vi "ATF Pumb-RT_Main.vi"   [LabVIEW 2022 SP3]
uses:
  RT Controls/RT main.ctl
  RT Support/SeCrTs-RT_Global_R.vi
panel:
  # "RT main ATF-Pump"
types:
  T1 = typedef "RT main.ctl" = enum16{"initialise", "Wait for connection", "Wait for command"}
  T2 = enum16{"Init", "Read 'All'", "Read 'n'", "Read '1'", "Write '1'", "Write 'n'", "Write 'All'"}
  T3 = cluster{"Drive Control":cluster{"En_Drive_A":bool, "En_Drive_L":bool, "Exit_Drive_A":bool, "Exit_Drive_L":bool}, "Drive_ATF Control":cluster{"S.Freq":dbl, "Ramp up Time":dbl, "Ramp down Time":dbl, "Drive Speed":dbl, "Drive condition":dbl}, "Drive_LOX Control":cluster{"S.Freq":dbl, "Ramp up Time":dbl, "Ramp down Time":dbl, "Drive Speed":dbl, "Drive condition":dbl}, "Aconnection ID":refnum<k5>, "Lconnection ID":refnum<k5>, "Loop Control":cluster{"Start DAQ":bool, "Stop DAQ":bool, "RT Stop":bool, "RT Exit":bool, "Start Seq":bool}}
  T4 = typedef "SeCrTs-Data FIFO.ctl" = cluster{"RD":cluster{"AI_V_Data RD":refnum<queue>, "AI_C_Data RD":refnum<queue>, "AO_Data RD":refnum<queue>, "DI_Data RD":refnum<queue>, "ACC_Data RD":refnum<queue>, "TC_Data RD":refnum<queue>, "Drive_A_C RD":refnum<queue>, "Drive_A_D RD":refnum<queue>, "Drive_L_C RD":refnum<queue>, "Drive_L_D RD":refnum<queue>, "DI Data":refnum<queue>, "DO_Data RD":refnum<queue>}, "Err Pump":refnum<queue>}
  T5 = cluster{"Device List":cluster{"AO Cards":tag[], "AI Cards":tag[], "DI Cards":tag[], "DO Cards":tag[]}, "Channel List":cluster{"AI Channel list":tag[], "AO Channel list":tag[], "DO Channel list ":tag[], "DI Channel list":tag[]}}
  T6 = cluster{cluster{"Sr. No.":string, "Time CDT":string, "Component ID":string, "Data Type":string, "Condition":string, "Range/Position":string, "No of Samples for Pass":string, "Event Duration":string, "Continuous /Cumulative":string, "Expected Delay":string, "Failure case Seq":string, "Current Sequence":string}[]}[]
  T7 = cluster{"AO config":cluster{"Channel_Name":string, "Channel_Number":string, "Default_Value":dbl, "Units":string}[], "AI config":cluster{"Channel_Name":string, "Channel_Number":string, "Pre_Scale_min":dbl, "Pre_Scale_max":dbl, "Sensor_min":dbl, "Sensor_max":dbl, "Units":string}[], "DI config":cluster{"Channel_Name":string, "Channel_Number":string, "Default_Value":bool, "DI invert?":bool}[], "DO config":cluster{"Channel_Name":string, "Channel_Number":string, "Default_Value":bool, "DO invert?":bool}[], "TC config":cluster{"Channel_Name":string, "Channel_Number":string, "Pre_Scale_min":dbl, "Pre_Scale_max":dbl, "units":i32, " type":i32}[], "ACC config":cluster{"Channel_Name":string, "Channel_Number":string, "Pre_Scale_min":dbl, "Pre_Scale_max":dbl, "Terminal configuration":i32, "Sensitivity":dbl, "Sensitivity units":i32}[], "SG config":cluster{"Channel_Name":string, "Channel_Number":string, "Pre_Scale_min":dbl, "Pre_Scale_max":dbl}[], "Strain Gauge Settings":cluster{"poisson ratio":dbl, "nominal gage resistance":dbl, "gage factor":dbl}, "Bridge Settings":cluster{"voltage excitation value":dbl, "voltage excitation source":i32, "initial bridge voltage":dbl, "lead wire resistance":dbl, "strain configuration":i32}, "Sample Rate":cluster{"AI Sample Rate":dbl[], "AO Sample Rate":dbl[], "DI Sample Rate":dbl[], "TC Sample Rate":dbl[], "DO Sample Rate":dbl[], "SG Sample Rate":dbl[], "ACC Sample Rate":dbl[]}}
  T8 = enum16{"Init", "Read", "Write 'All'", "Write 'n'", "Write Safe Value", "Write Start Time", "Overwrite Pattern", "Overwrite Pattern with Start", "Append Pattern", "Start Pattern Mode", "Abort Pattern Mode", "Read 1"}
  T9 = cluster{"S.Freq":dbl, "Ramp up Time":dbl, "Ramp down Time":dbl, "Drive Speed":dbl, "Drive condition":dbl}
  T10 = cluster{"AO Cards":tag[], "AI Cards":tag[], "DI Cards":tag[], "DO Cards":tag[]}
  T11 = cluster{"AI Channel list":tag[], "AO Channel list":tag[], "DO Channel list ":tag[], "DI Channel list":tag[]}
  T12 = cluster{"Start DAQ":bool, "Stop DAQ":bool, "RT Stop":bool, "RT Exit":bool, "Start Seq":bool}
  T13 = cluster{"En_Drive_A":bool, "En_Drive_L":bool, "Exit_Drive_A":bool, "Exit_Drive_L":bool}
  T14 = cluster{"Manual HOLD":bool, "Automatic Hold AI":bool, "Abort":bool, "Automatic Hold DI":bool}
  T15 = cluster{"Channel_Name":string, "Channel_Number":string, "Default_Value":bool, "DO invert?":bool}[]
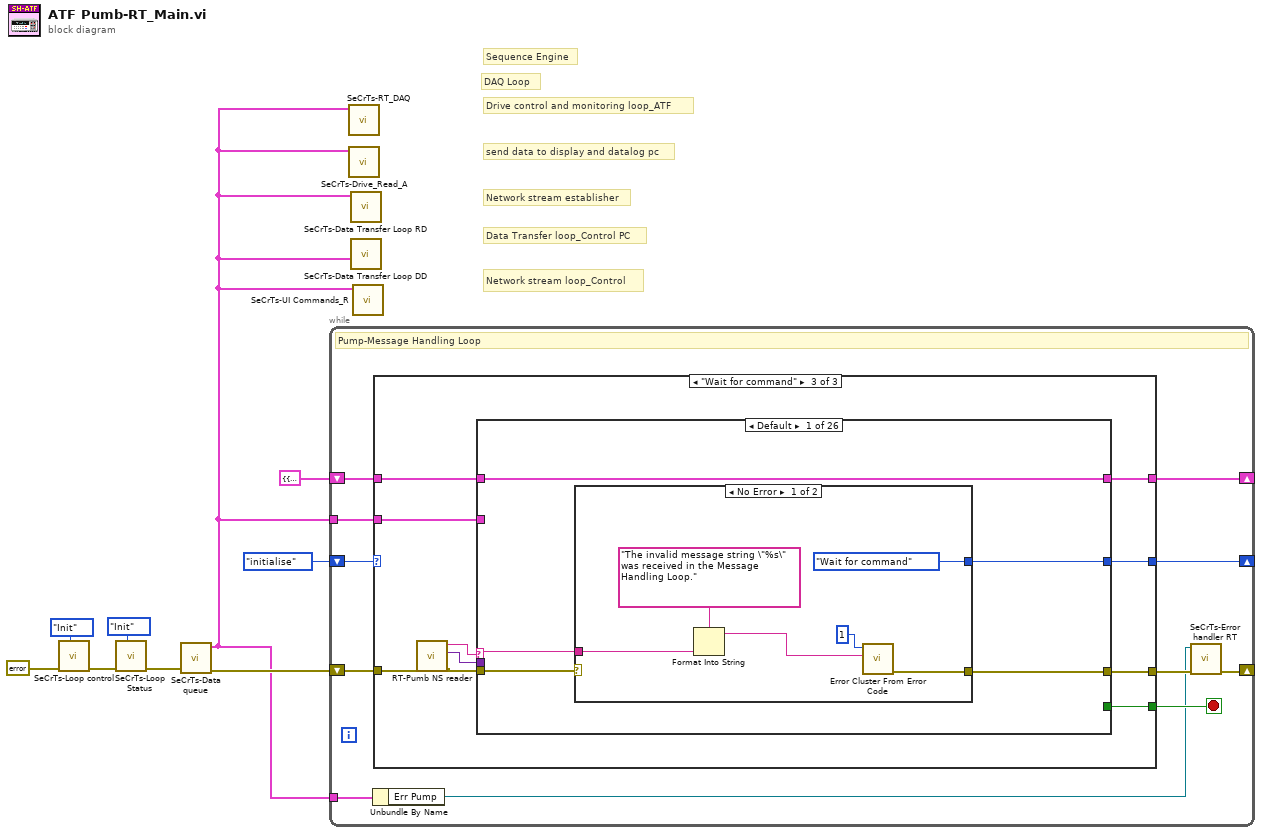
[diagram p0: block diagram]
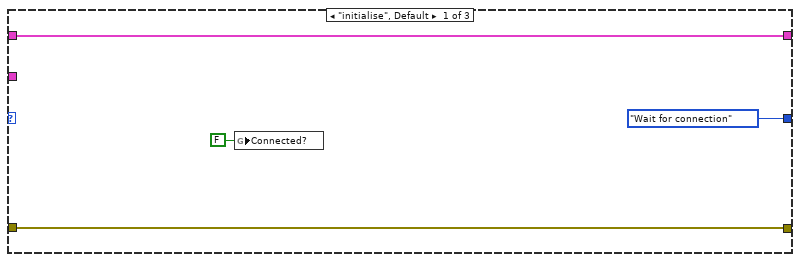
[diagram p2: hidden frame]
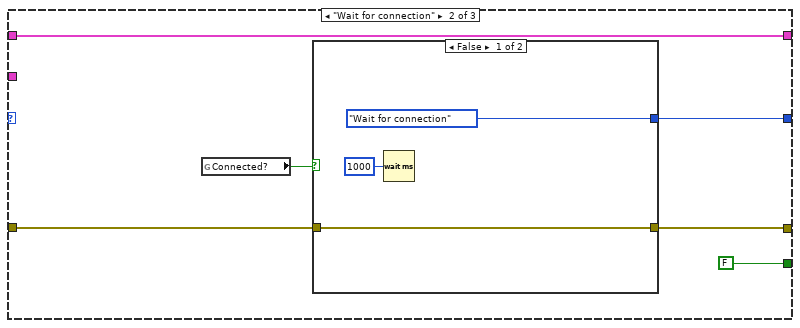
[diagram p3: hidden frame]
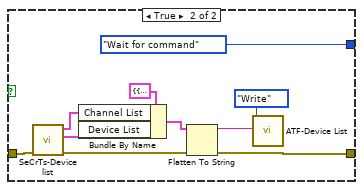
[diagram p4: hidden frame]
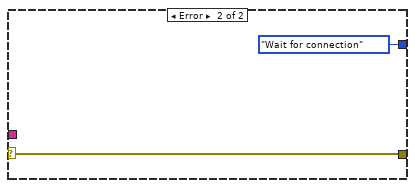
[diagram p5: hidden frame]
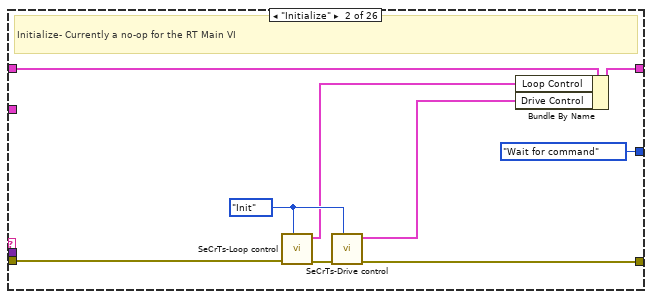
[diagram p6: hidden frame]
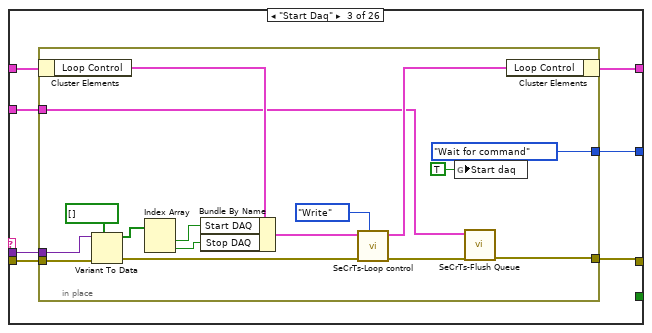
[diagram p7: hidden frame]
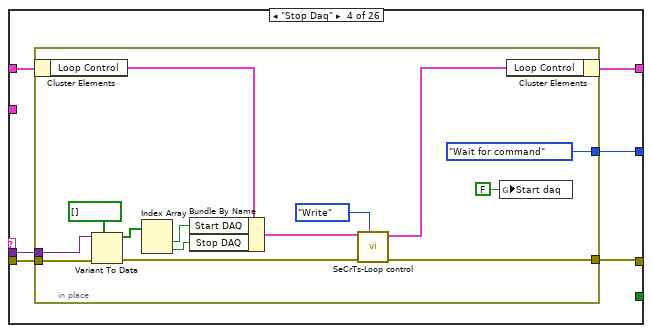
[diagram p8: hidden frame]
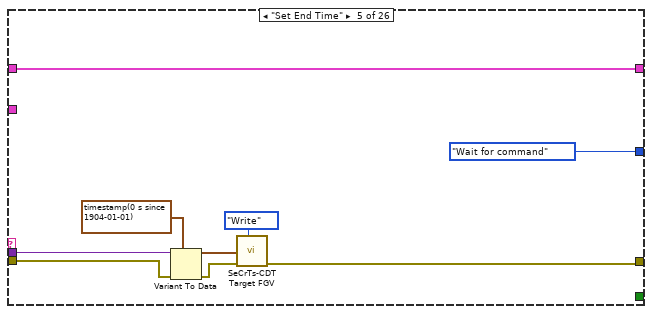
[diagram p9: hidden frame]
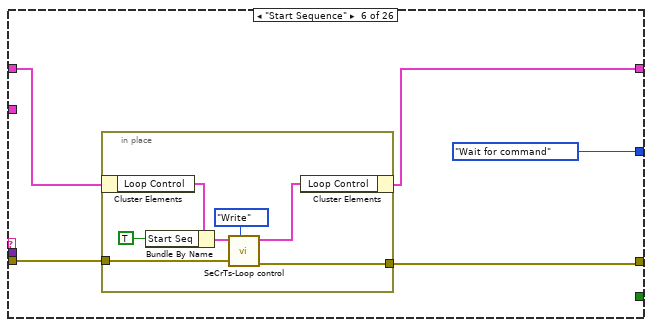
[diagram p10: hidden frame]
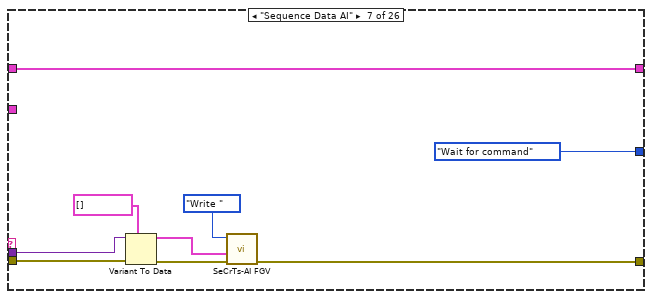
[diagram p11: hidden frame]
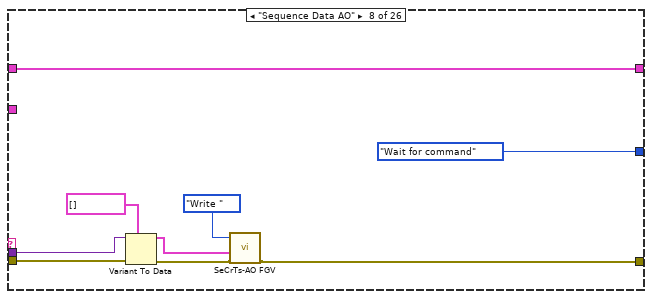
[diagram p12: hidden frame]
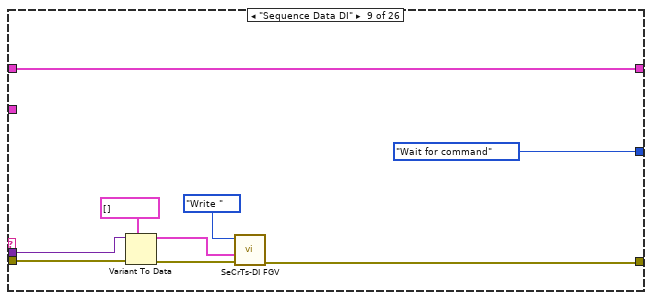
[diagram p13: hidden frame]
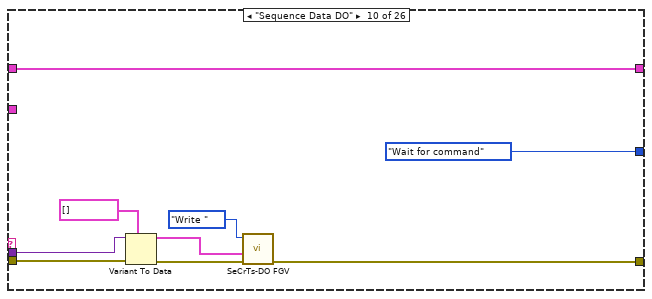
[diagram p14: hidden frame]
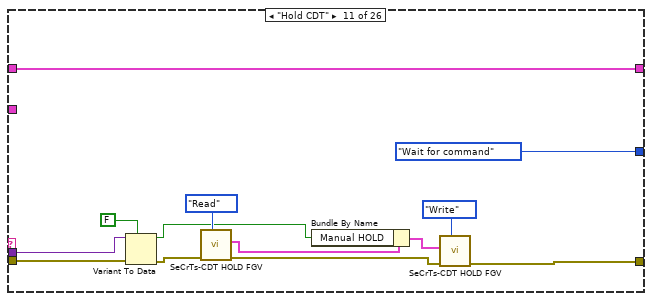
[diagram p15: hidden frame]
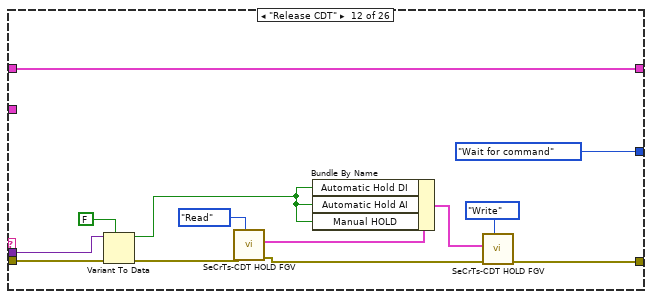
[diagram p16: hidden frame]
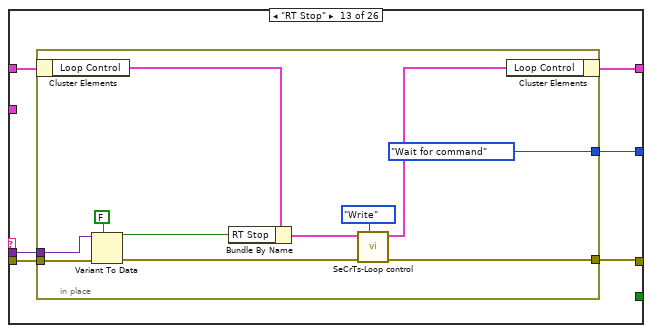
[diagram p17: hidden frame]
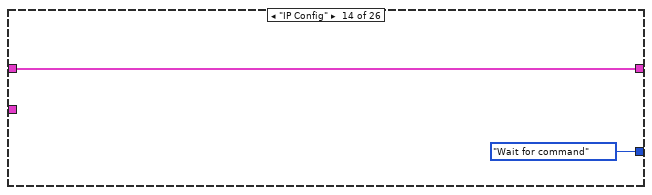
[diagram p18: hidden frame]
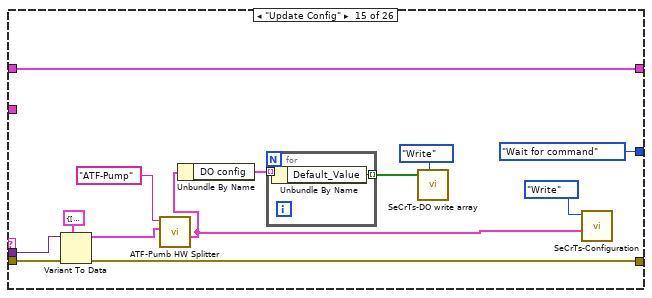
[diagram p19: hidden frame]
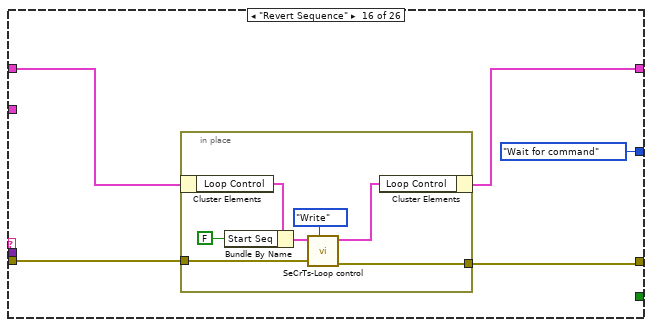
[diagram p20: hidden frame]
diagram:
  # "Sequence Engine"
  # "send data to display and datalog pc"
  # "Network stream establisher"
  # "Data Transfer loop_Control PC"
  # "Drive control and monitoring loop_ATF"
  # "DAQ Loop"
  # "Network stream loop_Control"
  n1 = call "SeCrTs-Loop control.vi"("Action"=enum16{"Init", "Write", "Read"}."Init", "error in (no error)"=errorcluster {"status"=FALSE, "code"=0, "source"=""} ("error constant")) -> ("error Out"=w4:errorcluster)  [unwired: 8 in, 1 out]
  n2 = call "SeCrTs-Loop Status.vi"("Option"=T2."Init", "error in (no error)"=w4) -> ("error out"=w7:errorcluster)  [unwired: 7 in, 2 out]
  n3 = call "SeCrTs-Data queue.vi"("error in"=w7) -> ("Data FIFO Ref"=w2:T4, "error out"=w3:errorcluster)  [unwired: 8 in]
  n4 = while {
    shift-right: [w15] -> _
    shift-left: w3 -> [w20]
    shift-right: [w17] -> _
    shift-left: T3 {"Drive Control"={"En_Drive_A"=FALSE, "En_Drive_L"=FALSE, "Exit_Drive_A"=FALSE, "Exit_Drive_L"=FALSE}, "Drive_ATF Control"={"S.Freq"=0.0, "Ramp up Time"=0.0, "Ramp down Time"=0.0, "Drive Speed"=0.0, "Drive condition"=0.0}, "Drive_LOX Control"={"S.Freq"=0.0, "Ramp up Time"=0.0, "Ramp down Time"=0.0, "Drive Speed"=0.0, "Drive condition"=0.0}, "Aconnection ID"=refnum, "Lconnection ID"=refnum, "Loop Control"={"Start DAQ"=FALSE, "Stop DAQ"=FALSE, "RT Stop"=FALSE, "RT Exit"=FALSE, "Start Seq"=FALSE}} -> [w18]
    tunnel: w2 -> [w14]
    tunnel: w2 -> [w13]
    shift-right: [w10] -> _
    shift-left: RT_main."initialise" ("Enum") -> [w11]
    stop <- w19 stop-if-true
    # "Pump-Message Handling Loop"
    n5 = Unbundle By Name(w13) -> ("Err Pump"=w12:refnum<queue>)
    n6 = case shown="\"Wait for command\"" w11 {
      tunnel: w20 -> [w21 w29 w48]
      tunnel: [_ FALSE w53] -> w19
      tunnel: w18 -> [w22 w25 w52]
      tunnel: [w22 w25 w51] -> w17
      tunnel: [w21 w28 w50] -> w16
      tunnel: w14 -> [_ _ w49]
      tunnel: [RT_main."Wait for connection" ("Enum") w27 w44] -> w10
      frame "initialise", Default {
        n7 = global write "SeCrTs-RT_Global_R.vi" "Connected?"(FALSE ("Connected?")) -> ()
      }
      frame "Wait for connection" {
        n8 = global read "SeCrTs-RT_Global_R.vi" "Connected?"() -> (w30:bool)
        n9 = case shown="False" w30 {
          tunnel: w29 -> [w33 w36]
          tunnel: [w33 w35] -> w28
          tunnel: [RT_main."Wait for connection" ("Enum") RT_main."Wait for command" ("Enum")] -> w27
          frame False {
            n10 = Wait (ms)(milliseconds to wait=u32 1000) -> ()  [unwired: 1 out]
          }
          frame True {
            n11 = call "SeCrTs-Device list.vi"("error in (no error)"=w36) -> ("error out"=w34:errorcluster, "Device List"=w40:T10, "Channel List"=w41:T11)  [unwired: 8 in]
            n12 = Bundle By Name(cluster=T5 {"Device List"={"AO Cards"=[], "AI Cards"=[], "DI Cards"=[], "DO Cards"=[]}, "Channel List"={"AI Channel list"=[], "AO Channel list"=[], "DO Channel list "=[], "DI Channel list"=[]}}, "Channel List"=w41, "Device List"=w40) -> (w39:T5)
            n13 = Flatten To String(anything=w39, error in (no error)=w34) -> (data string=w37:string, error out=w35:errorcluster)  [unwired: 2 in, 1 out]
            n14 = call "ATF-Device List.vi"("DL"=w37, "Enum"=enum16{"Write", "Read"}."Write") -> ()  [unwired: 8 in, 2 out]
          }
        }
      }
      frame "Wait for command" {
        n15 = call "RT-Pumb NS reader.vi"("error in (no error)"=w48) -> ("error IO"=w47:errorcluster, "Message Data"=w46:variant, "Message"=w45:string)  [unwired: 8 in]
        n16 = case shown="Default" w45 {
          selector: w45 -> [w57 _ _ _ _ _ _ _ _ _ _ _ _ _ _ _ _ _ _ _ _ _ _ _ _ _]
          tunnel: w46 -> [_ _ w80 w102 w126 _ w144 w155 w164 w173 w186 w196 w205 _ w230 _ w254 w260 w268 w284 w301 w327 w341 _ _ w360]
          tunnel: w47 -> [w55 w69 w82 w104 w125 w130 w146 w156 w165 w174 w187 w199 w207 _ w231 w238 w255 w262 w269 w285 w302 w328 w342 _ _ w361]
          tunnel: [w56 w68 w81 w103 w121 w131 w143 w153 w162 w172 w183 w198 w206 _ w225 w237 w251 _ w267 w283 w300 w326 w340 _ _ w359] -> w50
          tunnel: [_ _ _ _ _ _ _ _ _ _ _ _ _ _ _ _ _ _ _ _ _ _ _ _ _ w358] -> w53
          tunnel: w52 -> [w58 w71 w79 w101 w127 w132 w148 w157 w166 w175 w188 w201 w204 w220 w233 w240 w256 w263 w266 w282 w299 w325 w339 w352 w354 w357]
          tunnel: [w58 w70 w78 w100 w127 w129 w148 w157 w166 w175 w188 w201 w203 w220 w233 w239 w256 w263 w265 _ w298 w324 w338 w352 w354 w356] -> w51
          tunnel: w49 -> [_ _ w77 _ _ _ _ _ _ _ _ _ _ _ _ _ _ _ _ _ _ _ _ _ _ _]
          tunnel: [w54 RT_main."Wait for command" ("Enum") w76 w99 RT_main."Wait for command" ("Enum") RT_main."Wait for command" ("Enum") RT_main."Wait for command" ("Enum") RT_main."Wait for command" ("Enum") RT_main."Wait for command" ("Enum") RT_main."Wait for command" ("Enum") RT_main."Wait for command" ("Enum") RT_main."Wait for command" ("Enum") w202 RT_main."Wait for command" ("Enum") RT_main."Wait for command" ("Enum") RT_main."Wait for command" ("Enum") RT_main."Wait for command" ("Enum") RT_main."Wait for command" ("Enum") w264 w281 w297 w323 w337 RT_main."Wait for command" ("Enum") RT_main."Wait for command" ("Enum") w355] -> w44
          frame Default {
            n17 = case shown="No Error" w55 {
              selector: w55 -> [_ w65]
              tunnel: w57 -> [w61 _]
              tunnel: [w60 w65] -> w56
              tunnel: [RT_main."Wait for command" ("Enum") RT_main."Wait for connection" ("Enum")] -> w54
              frame No Error {
                n18 = Format Into String(format string="The invalid message string \"%s\" was received in the Message Handling Loop." ("Unknown Message Error Text"), w61) -> (resulting string=w62:string)  [unwired: 2 in, 1 out]
                n19 = call <vilib>:"Error Cluster From Error Code.vi"("error message (\"\")"=w62, "error code (0)"=1) -> ("error out"=w60:errorcluster)  [unwired: 7 in]
              }
              frame Error {
              }
            }
          }
          frame "Initialize" {
            w74 = enum16{"Init", "Write", "Read"}."Init" ("Action")
            # "Initialize- Currently a no-op for the RT Main VI"
            n20 = call "SeCrTs-Loop control.vi"("Action"=w74, "error in (no error)"=w69) -> ("error Out"=w75:errorcluster, "Loop Control out"=w73:T12)  [unwired: 8 in]
            n21 = call "SeCrTs-Drive control.vi"("Action"=w74, "error in"=w75) -> ("error Out"=w68:errorcluster, "Loop Control Out"=w72:T13)  [unwired: 8 in]
            n22 = Bundle By Name(cluster=w71, "Loop Control"=w73, "Drive Control"=w72) -> (w70:T3)
          }
          frame "Start Daq" {
            n23 = in-place {
              in-place-border: w82 -> [w97]
              in-place-border: [w86] -> w81
              in-place-border: w80 -> [w94]
              in-place-border: w77 -> [w85]
              in-place-border: [RT_main."Wait for command" ("Enum")] -> w76
              n24 = in-place-cluster #1(w79) -> ("Loop Control"=w93:T12)
              n25 = Variant To Data(error in=w97, type=bool[] [], Variant=w94) -> (data=w90:bool[], error out=w95:errorcluster)
              n26 = Index Array(array=w90) -> (element #1=w89:bool, element #2=w88:bool)  [unwired: 2 in]
              n27 = Bundle By Name(cluster=w93, "Start DAQ"=w89, "Stop DAQ"=w88) -> (w92:T12)
              n28 = call "SeCrTs-Loop control.vi"("Action"=enum16{"Init", "Write", "Read"}."Write", "error in (no error)"=w95, "Loop Control In"=w92) -> ("error Out"=w87:errorcluster, "Loop Control out"=w91:T12)  [unwired: 7 in]
              n29 = global write "SeCrTs-RT_Global_R.vi" "Start daq"(TRUE ("Start daq")) -> ()
              n30 = call "SeCrTs-Flush Queue.vi"("error in (no error)"=w87, "Data FIFO Ref"=w85) -> ("error out"=w86:errorcluster)  [unwired: 9 in]
              n31 = in-place-cluster #1("Loop Control"=w91) -> (w78:T3)
            }
          }
          frame "Stop Daq" {
            n32 = in-place {
              in-place-border: w104 -> [w117]
              in-place-border: [w114] -> w103
              in-place-border: w102 -> [w113]
              in-place-border: [RT_main."Wait for command" ("Enum")] -> w99
              n33 = in-place-cluster #2(w101) -> ("Loop Control"=w112:T12)
              n34 = Variant To Data(error in=w117, type=bool[] [], Variant=w113) -> (data=w109:bool[], error out=w115:errorcluster)
              n35 = Index Array(array=w109) -> (element #1=w108:bool, element #2=w107:bool)  [unwired: 2 in]
              n36 = Bundle By Name(cluster=w112, "Start DAQ"=w108, "Stop DAQ"=w107) -> (w111:T12)
              n37 = call "SeCrTs-Loop control.vi"("Action"=enum16{"Init", "Write", "Read"}."Write", "error in (no error)"=w115, "Loop Control In"=w111) -> ("error Out"=w114:errorcluster, "Loop Control out"=w110:T12)  [unwired: 7 in]
              n38 = global write "SeCrTs-RT_Global_R.vi" "Start daq"(FALSE ("Start daq")) -> ()
              n39 = in-place-cluster #2("Loop Control"=w110) -> (w100:T3)
            }
          }
          frame "Set End Time" {
            n40 = Variant To Data(error in=w125, type=timestamp(0 s since 1904-01-01) ("current time"), Variant=w126) -> (data=w123:timestamp, error out=w122:errorcluster)
            n41 = call "SeCrTs-CDT Target FGV.vi"("Enum"=enum16{"Write", "Read", "Init"}."Write", "error in"=w122, "Time Stamp"=w123) -> ("error out"=w121:errorcluster)  [unwired: 7 in, 1 out]
          }
          frame "Start Sequence" {
            n42 = in-place {
              in-place-border: w130 -> [w134]
              in-place-border: [w133] -> w131
              n43 = in-place-cluster #3(w132) -> ("Loop Control"=w139:T12)
              n44 = Bundle By Name(cluster=w139, "Start Seq"=TRUE ("Start DAQ")) -> (w136:T12)
              n45 = call "SeCrTs-Loop control.vi"("Action"=enum16{"Init", "Write", "Read"}."Write", "error in (no error)"=w134, "Loop Control In"=w136) -> ("error Out"=w133:errorcluster, "Loop Control out"=w135:T12)  [unwired: 7 in]
              n46 = in-place-cluster #3("Loop Control"=w135) -> (w129:T3)
            }
          }
          frame "Sequence Data AI" {
            n47 = Variant To Data(error in=w146, type=T6 [] ("Array"), Variant=w144) -> (data=w142:T6, error out=w145:errorcluster)
            n48 = call "SeCrTs-AI FGV.vi"("error in"=w145, "AI Seq  IN"=w142, "Enum"=enum16{"Read", "Write "}."Write ") -> ("error out"=w143:errorcluster)  [unwired: 7 in, 1 out]
          }
          frame "Sequence Data AO" {
            n49 = Variant To Data(error in=w156, type=T6 [] ("Array"), Variant=w155) -> (data=w152:T6, error out=w154:errorcluster)
            n50 = call "SeCrTs-AO FGV.vi"("error in"=w154, "AO Seq  IN"=w152, "Enum"=enum16{"Read", "Write "}."Write ") -> ("error out"=w153:errorcluster)  [unwired: 7 in, 1 out]
          }
          frame "Sequence Data DI" {
            n51 = Variant To Data(error in=w165, type=T6 [] ("Array"), Variant=w164) -> (data=w159:T6, error out=w163:errorcluster)
            n52 = call "SeCrTs-DI FGV.vi"("error in"=w163, "DI Seq  IN"=w159, "Enum"=enum16{"Read", "Write "}."Write ") -> ("error out"=w162:errorcluster)  [unwired: 7 in, 1 out]
          }
          frame "Sequence Data DO" {
            n53 = Variant To Data(error in=w174, type=T6 [] ("Array"), Variant=w173) -> (data=w168:T6, error out=w171:errorcluster)
            n54 = call "SeCrTs-DO FGV.vi"("error in"=w171, "DO Seq  IN"=w168, "Enum"=enum16{"Read", "Write "}."Write ") -> ("error out"=w172:errorcluster)  [unwired: 7 in, 1 out]
          }
          frame "Hold CDT" {
            n55 = Variant To Data(error in=w187, type=FALSE, Variant=w186) -> (data=w177:bool, error out=w181:errorcluster)
            n56 = call "SeCrTs-CDT HOLD FGV.vi"("Write/Read"=enum16{"Write", "Read"}."Read", "error in (no error)"=w181) -> ("error Out"=w180:errorcluster, "HOLD and Abort Out"=w178:T14)  [unwired: 6 in]
            n57 = Bundle By Name(cluster=w178, "Manual HOLD"=w177) -> (w179:T14)
            n58 = call "SeCrTs-CDT HOLD FGV.vi"("Write/Read"=enum16{"Write", "Read"}."Write", "error in (no error)"=w180, "HOLD and Abort"=w179) -> ("error Out"=w183:errorcluster)  [unwired: 5 in, 1 out]
          }
          frame "Release CDT" {
            n59 = Variant To Data(error in=w199, type=FALSE, Variant=w196) -> (data=w191:bool, error out=w190:errorcluster)
            n60 = call "SeCrTs-CDT HOLD FGV.vi"("Write/Read"=enum16{"Write", "Read"}."Read", "error in (no error)"=w190) -> ("error Out"=w193:errorcluster, "HOLD and Abort Out"=w194:T14)  [unwired: 6 in]
            n61 = Bundle By Name(cluster=w194, "Automatic Hold DI"=w191, "Automatic Hold AI"=w191, "Manual HOLD"=w191) -> (w192:T14)
            n62 = call "SeCrTs-CDT HOLD FGV.vi"("Write/Read"=enum16{"Write", "Read"}."Write", "error in (no error)"=w193, "HOLD and Abort"=w192) -> ("error Out"=w198:errorcluster)  [unwired: 5 in, 1 out]
          }
          frame "RT Stop" {
            n63 = in-place {
              in-place-border: w207 -> [w217]
              in-place-border: [w213] -> w206
              in-place-border: w205 -> [w212]
              in-place-border: [RT_main."Wait for command" ("Enum")] -> w202
              n64 = in-place-cluster #4(w204) -> ("Loop Control"=w211:T12)
              n65 = Variant To Data(error in=w217, type=FALSE, Variant=w212) -> (data=w216:bool, error out=w214:errorcluster)
              n66 = Bundle By Name(cluster=w211, "RT Stop"=w216) -> (w209:T12)
              n67 = call "SeCrTs-Loop control.vi"("Action"=enum16{"Init", "Write", "Read"}."Write", "error in (no error)"=w214, "Loop Control In"=w209) -> ("error Out"=w213:errorcluster, "Loop Control out"=w210:T12)  [unwired: 7 in]
              n68 = in-place-cluster #4("Loop Control"=w210) -> (w203:T3)
            }
          }
          frame "IP Config" {
          }
          frame "Update Config" {
            n69 = Variant To Data(error in=w231, type=T7 {"AO config"=[], "AI config"=[], "DI config"=[], "DO config"=[], "TC config"=[{"Channel_Name"="", "Channel_Number"="", "Pre_Scale_min"=0.0, "Pre_Scale_max"=0.0, "units"=4, " type"=7}], "ACC config"=[], "SG config"=[], "Strain Gauge Settings"={"poisson ratio"=0.3, "nominal gage resistance"=120.0, "gage factor"=2.08}, "Bridge Settings"={"voltage excitation value"=3.3, "voltage excitation source"=10200, "initial bridge voltage"=0.0, "lead wire resistance"=1.7, "strain configuration"=10271}, "Sample Rate"={"AI Sample Rate"=[], "AO Sample Rate"=[], "DI Sample Rate"=[], "TC Sample Rate"=[], "DO Sample Rate"=[], "SG Sample Rate"=[], "ACC Sample Rate"=[]}} ("Config in"), Variant=w230) -> (data=w224:T7, error out=w225:errorcluster)
            n70 = call "ATF-Pumb HW Splitter.vi"("data"=w224, "Pumb Expression"="ATF-Pump") -> ("Pumb HW"=w222:T7)  [unwired: 8 in, 1 out]
            n71 = Unbundle By Name(w222) -> ("DO config"=w227:T15)
            n72 = for {
              tunnel: w227 -> [w235] mode=indexing
              tunnel: [w234] -> w226 mode=indexing
              n73 = Unbundle By Name(w235) -> ("Default_Value"=w234:bool)
            }
            n74 = call "SeCrTs-DO write array.vi"("Enum"=enum16{"Write", "Read"}."Write", "DO Array"=w226) -> ()  [unwired: 9 in, 1 out]
            n75 = call "SeCrTs-Configuration.vi"("Config in"=w222, "Enum"=enum16{"Write", "Read"}."Write") -> ()  [unwired: 9 in, 1 out]
          }
          frame "Revert Sequence" {
            n76 = in-place {
              in-place-border: w238 -> [w242]
              in-place-border: [w241] -> w237
              n77 = in-place-cluster #5(w240) -> ("Loop Control"=w247:T12)
              n78 = Bundle By Name(cluster=w247, "Start Seq"=FALSE ("Start DAQ")) -> (w244:T12)
              n79 = call "SeCrTs-Loop control.vi"("Action"=enum16{"Init", "Write", "Read"}."Write", "error in (no error)"=w242, "Loop Control In"=w244) -> ("error Out"=w241:errorcluster, "Loop Control out"=w243:T12)  [unwired: 7 in]
              n80 = in-place-cluster #5("Loop Control"=w243) -> (w239:T3)
            }
          }
          frame "Write DO" {
            n81 = Variant To Data(error in=w255, type=bool[] [] ("DO Array"), Variant=w254) -> (data=w250:bool[], error out=w252:errorcluster)
            n82 = call "SeCrTs-DO Data FGV.vi"("DO Values In"=w250, "Option"=T8."Write 'All'", "error in (no error)"=w252) -> ("error out"=w251:errorcluster)  [unwired: 6 in, 6 out]
          }
          frame "Update Valve State" {
            n83 = Variant To Data(error in=w262, type=bool[] [], Variant=w260) -> (data=w259:bool[])  [unwired: 1 out]
            n84 = call "SeCrTs-DO Data FGV.vi"("DO Values In"=w259, "Option"=T8."Write Safe Value") -> ()  [unwired: 7 in, 7 out]
          }
          frame "Connect Drive ATF" {
            n85 = in-place {
              in-place-border: w269 -> [w279]
              in-place-border: w268 -> [w278]
              in-place-border: [w274] -> w267
              in-place-border: [RT_main."Wait for command" ("Enum")] -> w264
              n86 = in-place-cluster #6(w266) -> ("Drive Control"=w273:T13)
              n87 = Variant To Data(error in=w279, type=FALSE, Variant=w278) -> (data=w277:bool, error out=w275:errorcluster)
              n88 = Bundle By Name(cluster=w273, "En_Drive_A"=w277) -> (w272:T13)
              n89 = call "SeCrTs-Drive control.vi"("Action"=enum16{"Init", "Write", "Read"}."Write", "error in"=w275, "Loop Control In"=w272) -> ("error Out"=w274:errorcluster, "Loop Control Out"=w271:T13)  [unwired: 7 in]
              n90 = in-place-cluster #6("Drive Control"=w271) -> (w265:T3)
            }
          }
          frame "Exit Drive ATF" {
            n91 = in-place {
              in-place-border: w285 -> [w295]
              in-place-border: w284 -> [w294]
              in-place-border: [w289] -> w283
              in-place-border: [RT_main."Wait for command" ("Enum")] -> w281
              n92 = in-place-cluster #7(w282) -> ("Drive Control"=w288:T13)
              n93 = Variant To Data(error in=w295, type=FALSE, Variant=w294) -> (data=w293:bool, error out=w290:errorcluster)
              n94 = Bundle By Name(cluster=w288, "Exit_Drive_A"=w293) -> (w292:T13)
              n95 = call "SeCrTs-Drive control.vi"("Action"=enum16{"Init", "Write", "Read"}."Write", "error in"=w290, "Loop Control In"=w292) -> ("error Out"=w289:errorcluster, "Loop Control Out"=w287:T13)  [unwired: 7 in]
              n96 = in-place-cluster #7("Drive Control"=w287) -> ()  [unwired: 1 out]
            }
          }
          frame "Update Drive ATF" {
            n97 = in-place {
              in-place-border: w302 -> [w314]
              in-place-border: w301 -> [w313]
              in-place-border: [w308] -> w300
              in-place-border: [RT_main."Wait for command" ("Enum")] -> w297
              n98 = in-place-cluster #8(w299) -> ("Aconnection ID"=w305:refnum<k5>)
              n99 = Variant To Data(error in=w314, type=T9 {"S.Freq"=0.0, "Ramp up Time"=0.0, "Ramp down Time"=0.0, "Drive Speed"=0.0, "Drive condition"=0.0} ("Drive_ATF Control"), Variant=w313) -> (data=w312:T9, error out=w309:errorcluster)
              n100 = Cluster To Array(cluster=w312) -> (array=w311:dbl[])
              n101 = for {
                tunnel: w311 -> [w322] mode=indexing
                tunnel: i32[] [17, 18, 19, 20, 21] -> [w321] mode=indexing
                tunnel: [w320] -> w307 mode=indexing
                n102 = call "SeCrTs-Drive_Message.vi"("Input"=w322, "Packet \nIdentifier"=w321) -> ("String"=w320:string)  [unwired: 9 in]
              }
              n103 = for {
                tunnel: w307 -> [w317] mode=indexing
                shift-right: [w318] -> w308
                shift-left: w309 -> [w319]
                tunnel: w305 -> [w316]
                tunnel: [w315] -> w304
                n104 = TCP Write(connection ID=w316, data in=w317, error in (no error)=w319) -> (connection ID out=w315:refnum<k5>, error out=w318:errorcluster)  [unwired: 1 in, 1 out]
              }
              n105 = in-place-cluster #8("Aconnection ID"=w304) -> (w298:T3)
            }
          }
          frame "Motor On ATF" {
            n106 = in-place {
              in-place-border: w328 -> [w332]
              in-place-border: w327 -> [_]
              in-place-border: [w336] -> w326
              in-place-border: [RT_main."Wait for command" ("Enum")] -> w323
              n107 = in-place-cluster #9(w325) -> ("Aconnection ID"=w334:refnum<k5>)
              n108 = call "SeCrTs-Drive_Message.vi"("Input"=1.0, "Packet \nIdentifier"=17 ("Packet \nIdentifier")) -> ("String"=w335:string)  [unwired: 9 in]
              n109 = TCP Write(connection ID=w334, data in=w335, error in (no error)=w332) -> (connection ID out=w333:refnum<k5>, error out=w336:errorcluster)  [unwired: 1 in, 1 out]
              n110 = in-place-cluster #9("Aconnection ID"=w333) -> (w324:T3)
            }
          }
          frame "Motor Off ATF" {
            n111 = in-place {
              in-place-border: w342 -> [w346]
              in-place-border: w341 -> [_]
              in-place-border: [w350] -> w340
              in-place-border: [RT_main."Wait for command" ("Enum")] -> w337
              n112 = in-place-cluster #10(w339) -> ("Aconnection ID"=w348:refnum<k5>)
              n113 = call "SeCrTs-Drive_Message.vi"("Input"=0.0, "Packet \nIdentifier"=17 ("Packet \nIdentifier")) -> ("String"=w349:string)  [unwired: 9 in]
              n114 = TCP Write(connection ID=w348, data in=w349, error in (no error)=w346) -> (connection ID out=w347:refnum<k5>, error out=w350:errorcluster)  [unwired: 1 in, 1 out]
              n115 = in-place-cluster #10("Aconnection ID"=w347) -> (w338:T3)
            }
          }
          frame "Phase Code Update" {
          }
          frame "Abort" {
          }
          frame "RT Exit" {
            # "Initialize- Currently a no-op for the RT Main VI"
            n116 = in-place {
              in-place-border: w361 -> [w376]
              in-place-border: w360 -> [w374]
              in-place-border: [w371] -> w359
              in-place-border: [TRUE] -> w358
              in-place-border: [RT_main."Wait for command" ("Enum")] -> w355
              w370 = enum16{"Init", "Write", "Read"}."Write" ("Action")
              n117 = in-place-cluster #11(w357) -> ("Loop Control"=w368:T12, "Drive Control"=w367:T13)
              n118 = Variant To Data(error in=w376, type=FALSE, Variant=w374) -> (data=w373:bool, error out=w375:errorcluster)
              n119 = Bundle By Name(cluster=w367, "Exit_Drive_A"=w373) -> (w366:T13)
              n120 = Bundle By Name(cluster=w368, "RT Exit"=w373) -> (w365:T12)
              n121 = call "SeCrTs-Loop control.vi"("Action"=w370, "error in (no error)"=w375, "Loop Control In"=w365) -> ("error Out"=w372:errorcluster, "Loop Control out"=w363:T12)  [unwired: 7 in]
              n122 = call "SeCrTs-Drive control.vi"("Action"=w370, "error in"=w372, "Loop Control In"=w366) -> ("error Out"=w371:errorcluster, "Loop Control Out"=w364:T13)  [unwired: 7 in]
              n123 = in-place-cluster #11("Loop Control"=w363, "Drive Control"=w364) -> (w356:T3)
            }
          }
        }
      }
    }
    n124 = call "SeCrTs-Error handler RT.vi"("error in"=w16, "Message Queue"=w12) -> ("error out"=w15:errorcluster)  [unwired: 8 in, 1 out]
  }
  n125 = call "SeCrTs-RT_DAQ.vi"("Data FIFO Ref"=w2) -> ()  [unwired: 10 in, 1 out]
  n126 = call "SeCrTs-Drive_Read_A.vi"("Data FIFO Ref"=w2) -> ()  [unwired: 10 in, 1 out]
  n127 = call "SeCrTs-Data Transfer Loop RD.vi"("Data FIFO Ref"=w2) -> ()  [unwired: 11 in]
  n128 = call "SeCrTs-Data Transfer Loop DD.vi"("Data FIFO Ref"=w2) -> ()  [unwired: 11 in]
  n129 = call "SeCrTs-UI Commands_R.vi"("Data FIFO Ref"=w2) -> ()  [unwired: 11 in]
